vi "Close Fan Tasks.vi"(8 "Error In":errorcluster, 11 "Hellicopter Tasks Input 2":T1) -> (0 "Error Out":errorcluster)   [LabVIEW 2017]
uses:
  <vilib>/DAQmx/write.llb/DAQmx Write (Analog 1D DBL NChan 1Samp).vi
  <vilib>/DAQmx/miscellaneous.llb/DAQmx Fill In Error Info.vi
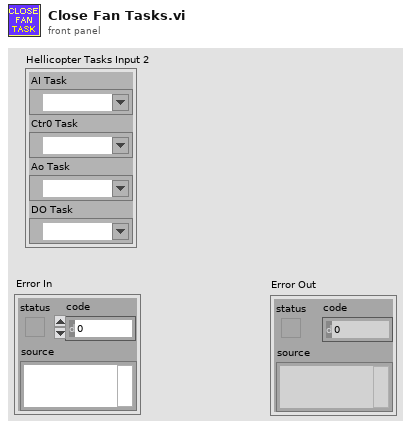
[diagram p1: front panel]
types:
  T1 = cluster{"AI Task":refnum<k21>, "Ctr0 Task":refnum<k21>, "Ao Task":refnum<k21>, "DO Task":refnum<k21>}
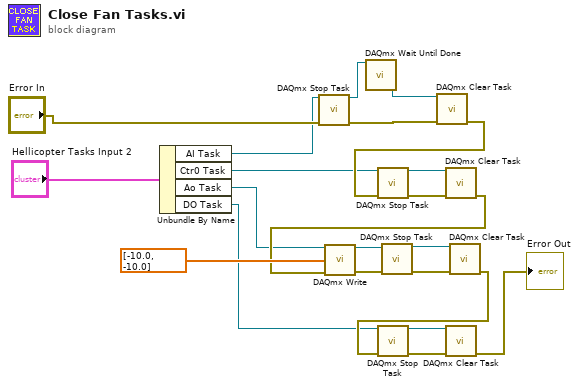
[diagram p0: block diagram]
diagram:
  n1 = Unbundle By Name("Hellicopter Tasks Input 2") -> ("AI Task"=w10:refnum<k21>, "Ctr0 Task"=w9:refnum<k21>, "Ao Task"=w8:refnum<k21>, "DO Task"=w3:refnum<k21>)
  n2 = call <vilib>:"DAQmx Stop Task.vi"("task/channels in"=w10, "error in"="Error In") -> ("task out"=w14:refnum<k21>, "error out"=w15:errorcluster)  [unwired: 12 in]
  n3 = call <vilib>:"DAQmx Wait Until Done.vi"("task/channels in"=w14) -> ("task out"=w1:refnum<k21>)  [unwired: 13 in, 1 out]
  n4 = call <vilib>:"DAQmx Clear Task.vi"("task in"=w1, "error in"=w15) -> ("error out"=w12:errorcluster)  [unwired: 13 in]
  n5 = call <vilib>:"DAQmx Stop Task.vi"("task/channels in"=w9, "error in"=w12) -> ("task out"=w17:refnum<k21>, "error out"=w16:errorcluster)  [unwired: 12 in]
  n6 = call <vilib>:"DAQmx Clear Task.vi"("task in"=w17, "error in"=w16) -> ("error out"=w13:errorcluster)  [unwired: 13 in]
  n7 = call-poly <vilib>:"DAQmx Write.vi"("task/channels in"=w8, "data"=dbl[] [-10.0, -10.0], "error in"=w13) -> ("task out"=w21:refnum<k21>, "error out"=w20:errorcluster)  [unwired: 10 in, 1 out]
  n8 = call <vilib>:"DAQmx Stop Task.vi"("task/channels in"=w21, "error in"=w20) -> ("task out"=w18:refnum<k21>, "error out"=w19:errorcluster)  [unwired: 12 in]
  n9 = call <vilib>:"DAQmx Clear Task.vi"("task in"=w18, "error in"=w19) -> ("error out"=w4:errorcluster)  [unwired: 13 in]
  n10 = call <vilib>:"DAQmx Stop Task.vi"("task/channels in"=w3, "error in"=w4) -> ("task out"=w2:refnum<k21>, "error out"=w6:errorcluster)  [unwired: 12 in]
  n11 = call <vilib>:"DAQmx Clear Task.vi"("task in"=w2, "error in"=w6) -> ("error out"=→"Error Out":errorcluster)  [unwired: 13 in]
